vi "Sea-Level SWI Ports to Array of States.vi"(2 "SWI Position":T1) -> (6 "Number of Ports":i8, 7 "State Array":bool[](array[boolean]))   [LabVIEW 2011]
uses:
  TypeDefs/Sea-Level SWI Position.ctl
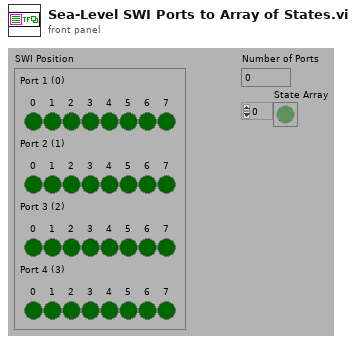
[diagram p1: front panel]
types:
  T1 = typedef "Sea-Level SWI Position.ctl" = cluster{"Port 1 (0)":cluster{"0":bool, "1":bool, "2":bool, "3":bool, "4":bool, "5":bool, "6":bool, "7":bool}, "Port 2 (1)":cluster{"0":bool, "1":bool, "2":bool, "3":bool, "4":bool, "5":bool, "6":bool, "7":bool}, "Port 3 (2)":cluster{"0":bool, "1":bool, "2":bool, "3":bool, "4":bool, "5":bool, "6":bool, "7":bool}, "Port 4 (3)":cluster{"0":bool, "1":bool, "2":bool, "3":bool, "4":bool, "5":bool, "6":bool, "7":bool}}
  T2 = cluster{"0":bool, "1":bool, "2":bool, "3":bool, "4":bool, "5":bool, "6":bool, "7":bool}[]
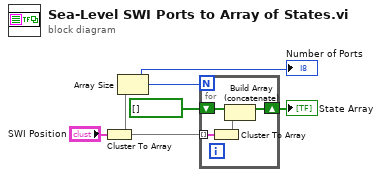
[diagram p0: block diagram]
diagram:
  n1 = Cluster To Array(cluster="SWI Position") -> (array=w4:T2)
  n2 = Array Size(array=w4) -> (size(s)=w3:i32)
  "Number of Ports" <- w3
  n3 = for {
    N: w3 -> [_]
    tunnel: w4 -> [w9] mode=indexing
    shift-right: [w7] -> w1
    shift-left: bool[] [] ("State Array") -> [w8]
    n4 = Cluster To Array(cluster=w9) -> (array=w6:bool[])
    n5 = Build Array (concatenate)(w8, w6) -> (w7:bool[])
  }
  "State Array" <- w1
